vi "IMAQ FPGA Image Transfer from Target U8.vi"(6 "Image Transfer Size Alignment":u32(ring)=1 items=["1 Pixel"=1, "8 Pixels"=8, "16 Pixels"=16, "32 Pixels"=32], 7 "Read Timeout (ms)":i32=5000, 8 "error in (no error)":errorcluster, 9 "DMA FIFO Reference In":refnum<k20>, 10 "Maximum Pixels per Read":i32=-1, 11 "Image":T1) -> (0 "error out":errorcluster, 1 "DMA FIFO Reference Out":refnum<k20>, 3 "Image Out":T1)   [LabVIEW 2020, in "NI_VDM_FPGA_Basics.lvlib"]
doc: "Transfers an image from the target FPGA to the host processor via DMA FIFO."
uses:
  <vilib>/visionFPGA/NI_VDM_FPGA_Basics.lvlib
  <vilib>/vision/Image Controls.llb/IMAQ Image.ctl
  <vilib>/rvi/errors/niLvFpgaAdjustHostInterfaceError.vi
  <vilib>/rvi/interface/nirviMethod/nirviMethod.xnode
  <vilib>/FPGAPlugInAG/Dynamic/niLvFpga_ReadFifo_Dynamic.vi
  <vilib>/rvi/errors/niLvFpgaMergeErrorWithErrorCode.vi
  <vilib>/vision/EDVR.llb/IMAQ ImageToEDVR 2D U8.vi
  <vilib>/FPGAPlugInAG/Dynamic/niLvFpga_AcquireReadRegionFifo_Dynamic.vi
  nivissvc.dll
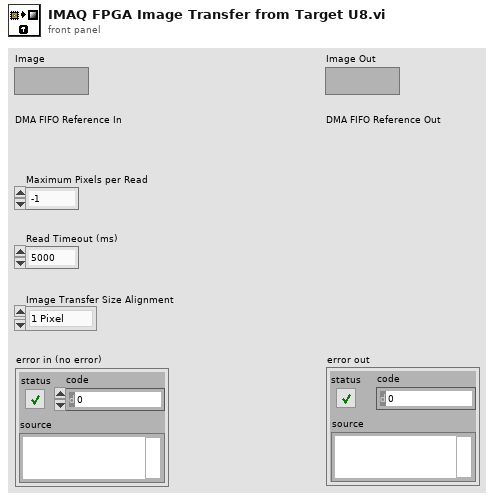
[diagram p1: front panel]
types:
  T1 = typedef "IMAQ Image.ctl" = refnum<image>
  T2 = typedef "Image Type" = u32
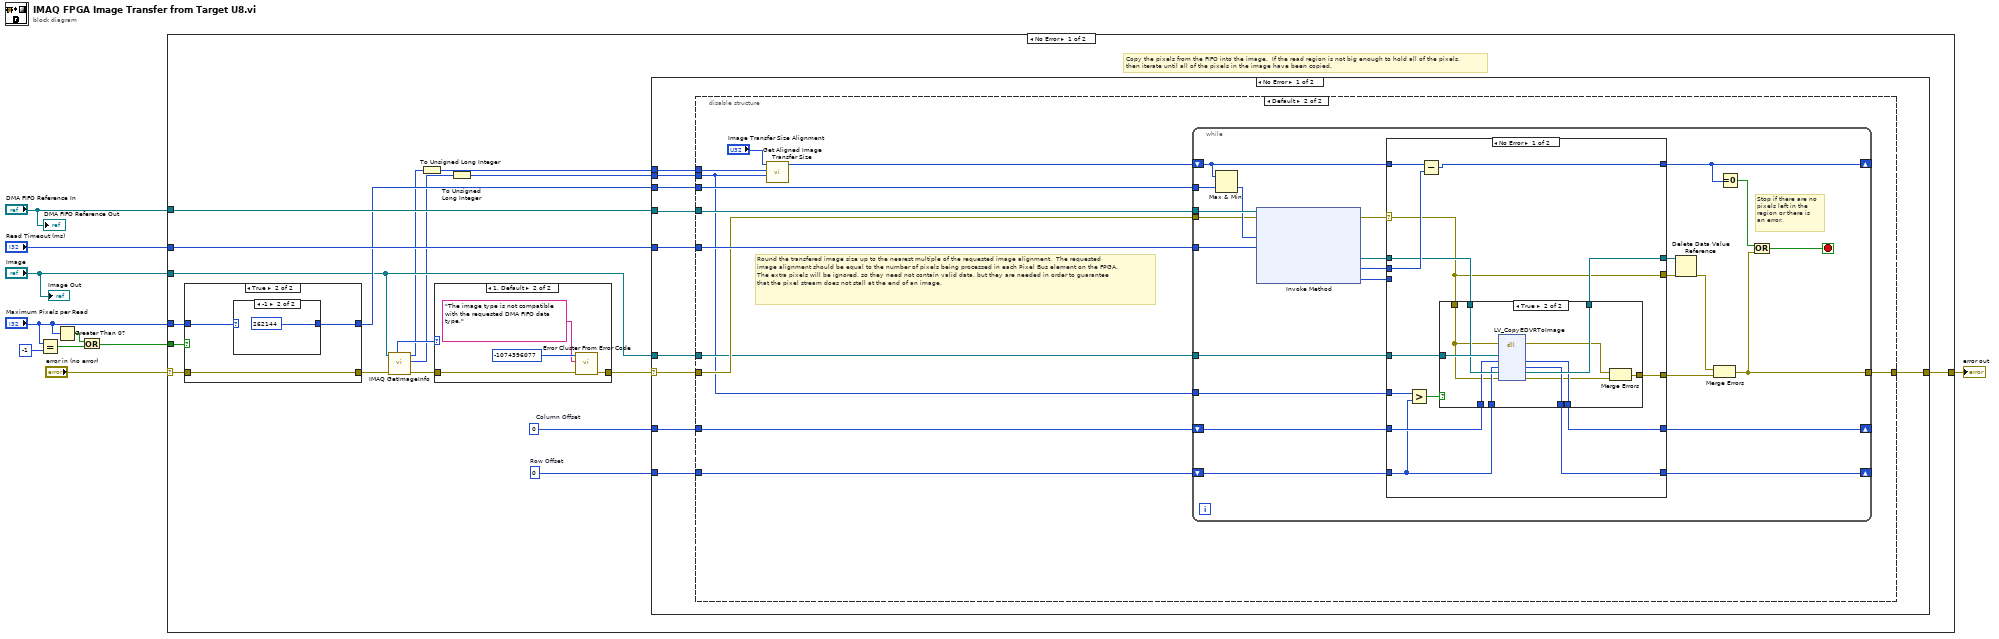
[diagram p0: block diagram]
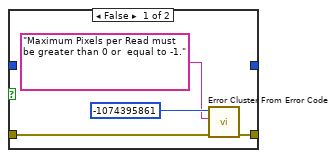
[diagram p2: hidden frame]
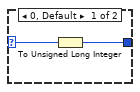
[diagram p3: hidden frame]
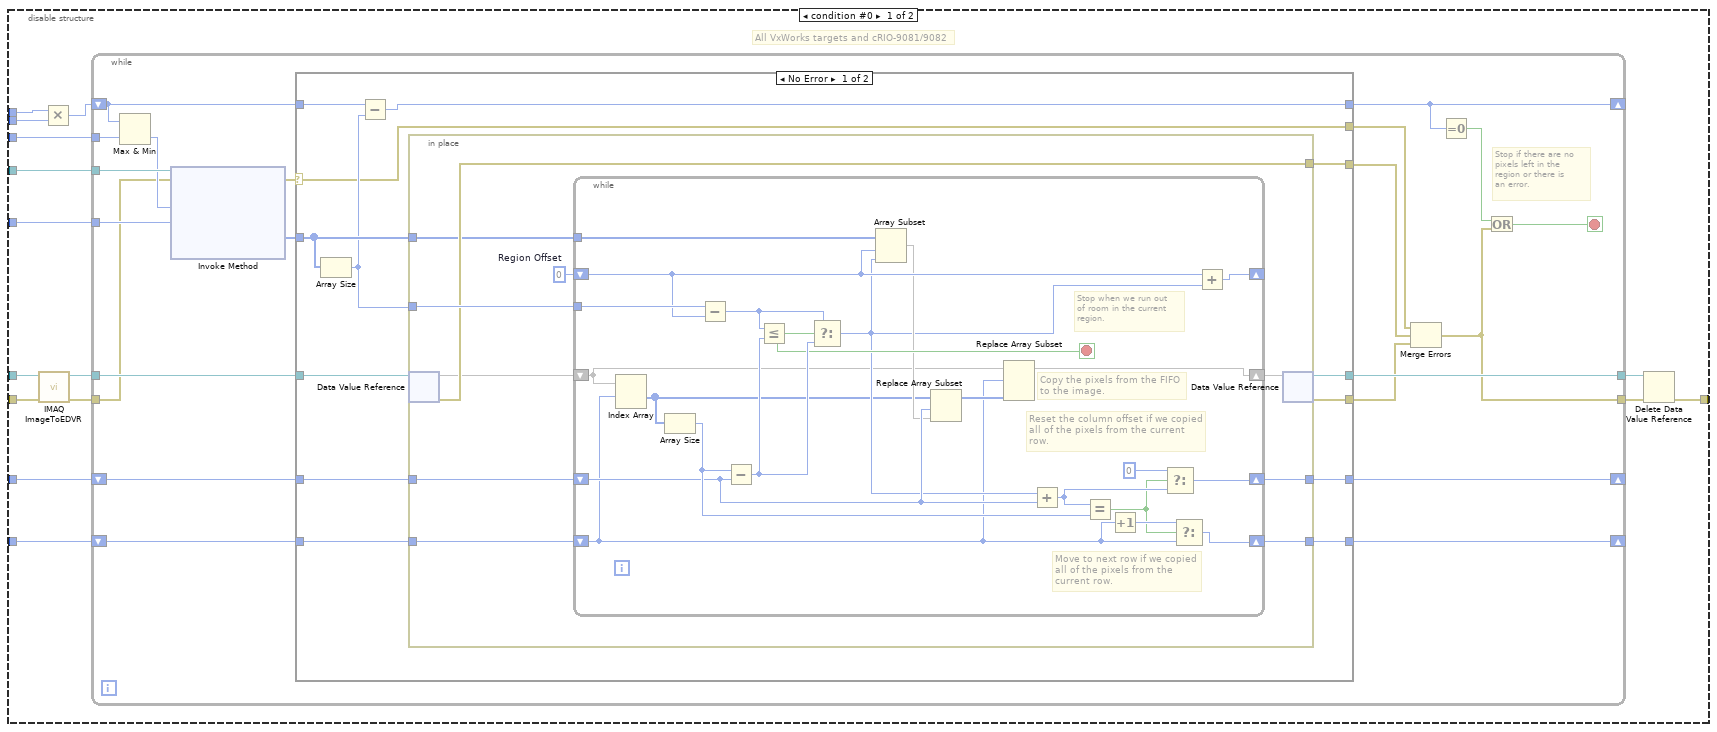
[diagram p5: hidden frame]
diagram:
  n1 = Equal?(x="Maximum Pixels per Read", y=-1) -> (x = y?=w6:bool)
  n2 = Greater Than 0?(x="Maximum Pixels per Read") -> (x > 0?=w7:bool)
  n3 = Or(x=w7, y=w6) -> (x .or. y?=w5:bool)
  n4 = case shown="No Error" "error in (no error)" {
    selector: "error in (no error)" -> [w15 w211]
    tunnel: "DMA FIFO Reference In" -> [w26 _]
    tunnel: "Read Timeout (ms)" -> [w23 _]
    tunnel: w5 -> [w22 _]
    tunnel: "Maximum Pixels per Read" -> [w21 _]
    tunnel: "Image" -> [w17 _]
    tunnel: [w16 w211] -> w2
    frame No Error {
      w27 = u32 0  # Row Offset
      w28 = u32 0  # Column Offset
      # "Copy the pixels from the FIFO into the image.  If the read region is not big enough to hold all of the pixels,\nthen iterate until all of the pixels in the image have been copied."
      n5 = case shown="True" w22 {
        tunnel: w15 -> [w30 w35]
        tunnel: [w29 w35] -> w20
        tunnel: w21 -> [_ w34]
        tunnel: [_ w33] -> w19
        frame False {
          n6 = call <vilib>:"Error Cluster From Error Code.vi"("error in (no error)"=w30, "error message (\"\")"="Maximum Pixels per Read must be greater than 0 or  equal to -1." ("error message (\"\")"), "error code (0)"=-1074395861) -> ("error out"=w29:errorcluster)  [unwired: 6 in]
        }
        frame True {
          n7 = case shown="-1" w34 {
            selector: w34 -> [w37 _]
            tunnel: [w36 u32 262144 ("Maximum Pixels per Write")] -> w33
            frame 0, Default {
              n8 = To Unsigned Long Integer(number=w37) -> (unsigned 32bit integer=w36:u32)
            }
            frame -1 {
            }
          }
        }
      }
      n9 = call "IMAQ GetImageInfo"("error in (no error)"=w20, "Image"=w17) -> ("error out"=w24:errorcluster, "Y Resolution"=w13:i32, "X Resolution"=w14:i32, "Image Type"=w25:T2)  [unwired: 2 in, 4 out]
      n10 = To Unsigned Long Integer(number=w14) -> (unsigned 32bit integer=w12:u32)
      n11 = case shown="1, Default" w25 {
        tunnel: w24 -> [w39 w41]
        tunnel: [w39 w40] -> w18
        frame 0 {
          # "Allowed types are:\nGrayscale (U8)"
        }
        frame 1, Default {
          n12 = call <vilib>:"Error Cluster From Error Code.vi"("error in (no error)"=w41, "error message (\"\")"="The image type is not compatible with the requested DMA FIFO data type." ("error message (\"\")"), "error code (0)"=-1074396077) -> ("error out"=w40:errorcluster)  [unwired: 6 in]
        }
      }
      n13 = To Unsigned Long Integer(number=w13) -> (unsigned 32bit integer=w11:u32)
      n14 = case shown="No Error" w18 {
        selector: w18 -> [w52 w210]
        tunnel: w28 -> [w51 _]
        tunnel: w27 -> [w50 _]
        tunnel: w26 -> [w48 _]
        tunnel: [w46 w210] -> w16
        tunnel: w19 -> [w47 _]
        tunnel: w23 -> [w49 _]
        tunnel: w17 -> [w53 _]
        tunnel: w12 -> [w45 _]
        tunnel: w11 -> [w44 _]
        frame No Error {
          n15 = disable-structure shown="Default" {
            disable-tunnel: w51 -> [w68 w151]
            disable-tunnel: w50 -> [w67 w150]
            disable-tunnel: w48 -> [w66 w149]
            disable-tunnel: [w57 w148] -> w46
            disable-tunnel: w47 -> [w65 w147]
            disable-tunnel: w49 -> [w64 w146]
            disable-tunnel: w53 -> [w63 w144]
            disable-tunnel: w52 -> [w61 w145]
            disable-tunnel: w45 -> [w55 w141]
            disable-tunnel: w44 -> [w54 w140]
            frame condition #0 {
              # "All VxWorks targets and cRIO-9081/9082"
              n16 = call-poly <vilib>:"IMAQ ImageToEDVR.vi"("error in (no error)"=w61, "Image"=w63) -> ("error out"=w60:errorcluster, "EDVR 2D U8"=w62:refnum<data-value>)  [unwired: 7 in, 1 out]
              n17 = Multiply(x=w55, y=w54) -> (x*y=w56:u32)
              n18 = while {
                shift-right: [w80] -> _
                shift-left: w56 -> [w76]
                shift-right: [w85] -> _
                shift-left: w68 -> [w87]
                shift-right: [w88] -> _
                shift-left: w67 -> [w86]
                tunnel: w66 -> [w84]
                tunnel: [w82] -> w59
                tunnel: [w78] -> w58
                tunnel: w65 -> [w74]
                tunnel: w64 -> [w73]
                tunnel: w62 -> [w70]
                tunnel: w60 -> [w69]
                stop <- w79 stop-if-true
                # "Stop if there are no\npixels left in the \nregion or there is\nan error."
                n19 = Max & Min(x=w76, y=w74) -> (min(x,y)=w75:u32)  [unwired: 1 out]
                n20 = xnode "Invoke Method"("FPGA VI Reference In"=w84, "error in"=w69, "Number of Elements"=w75, "Timeout (ms)"=w73) -> ("error out"=w83:errorcluster, "Data"=w89:u8[])  [unwired: 2 out]
                n21 = case shown="No Error" w83 {
                  selector: w83 -> [w90 w135]
                  tunnel: w76 -> [w102 w138]
                  tunnel: [w101 w138] -> w80
                  tunnel: w70 -> [w100 w139]
                  tunnel: w89 -> [w92 _]
                  tunnel: [w99 w136] -> w88
                  tunnel: w87 -> [w98 w137]
                  tunnel: w86 -> [w97 w136]
                  tunnel: [w96 w137] -> w85
                  tunnel: [w95 w139] -> w82
                  tunnel: [w90 w135] -> w72
                  tunnel: [w94 _] -> w71
                  tunnel: [w93 _] -> w81
                  frame No Error {
                    n22 = Array Size(array=w92) -> (size(s)=w91:i32)
                    n23 = Subtract(x=w102, y=w91) -> (x-y=w101:u32)
                    n24 = in-place {
                      in-place-border: w91 -> [w110]
                      in-place-border: [w112] -> w99
                      in-place-border: w98 -> [w109]
                      in-place-border: w97 -> [w105]
                      in-place-border: [w108] -> w96
                      in-place-border: [w107] -> w93
                      in-place-border: w92 -> [w103]
                      w111 = u32 0  # Region Offset
                      n25 = in-place-dvr #1(w100) -> (w106:u8[][], w107:errorcluster)
                      n26 = while {
                        shift-right: [w132] -> _
                        shift-left: w111 -> [w131]
                        tunnel: w103 -> [w121]
                        tunnel: w110 -> [w134]
                        shift-right: [w126] -> w108
                        shift-left: w109 -> [w122]
                        shift-right: [w113] -> w104
                        shift-left: w106 -> [w116]
                        shift-right: [w124] -> w112
                        shift-left: w105 -> [w114]
                        stop <- w123 stop-if-true
                        # "Stop when we run out\nof room in the current\nregion."
                        # "Copy the pixels from the FIFO\nto the image."
                        # "Reset the column offset if we copied\nall of the pixels from the current\nrow."
                        # "Move to next row if we copied\nall of the pixels from the\ncurrent row."
                        n27 = Index Array(array=w116, index (row)=w114) -> (element=w117:u8[])  [unwired: 1 in]
                        n28 = Array Size(array=w117) -> (size(s)=w130:i32)
                        n29 = Subtract(x=w134, y=w131) -> (x-y=w133:u32)
                        n30 = Subtract(x=w130, y=w122) -> (x-y=w129:u32)
                        n31 = Less Or Equal?(x=w133, y=w129) -> (x <= y?=w123:bool)
                        n32 = Select(t=w133, s=w123, f=w129) -> (s? t:f=w119:u32)
                        n33 = Array Subset(array=w121, index=w131, length=w119) -> (w120:u8[])
                        n34 = Replace Array Subset(array=w117, new element=w120, index=w122) -> (w115:u8[])
                        n35 = Replace Array Subset(array=w116, new element=w115, index (row)=w114) -> (w113:u8[][])  [unwired: 1 in]
                        n36 = Add(x=w119, y=w122) -> (x+y=w127:u32)
                        n37 = Equal?(x=w127, y=w130) -> (x = y?=w118:bool)
                        n38 = Increment(x=w114) -> (x+1=w125:u32)
                        n39 = Select(t=u32 0 ("Elements In Region"), s=w118, f=w127) -> (s? t:f=w126:u32)
                        n40 = Select(t=w125, s=w118, f=w114) -> (s? t:f=w124:u32)
                        n41 = Add(x=w131, y=w119) -> (x+y=w132:u32)
                      }
                      n42 = in-place-dvr #1(w104) -> (w95:refnum<data-value>, w94:errorcluster)
                    }
                  }
                  frame Error {
                  }
                }
                n43 = Merge Errors(w72, w81, w71) -> (w78:errorcluster)
                n44 = Equal To 0?(x=w80) -> (x = 0?=w77:bool)
                n45 = Or(x=w77, y=w78) -> (x .or. y?=w79:bool)
              }
              n46 = Delete Data Value Reference(data value reference=w59, error in=w58) -> (error out=w57:errorcluster)  [unwired: 1 out]
            }
            frame condition #1 (active) {
              # "Round the transfered image size up to the nearest multiple of the requested image alignment.  The requested image alignment should be equal to the number of pixels being processed in each Pixel Bus element on the FPGA.  The extra pixels will be ignored, so they need not contain valid data, but they are needed in order to guarantee that the pixel stream does not stall at the end of an image."
              n47 = call <vilib>:"Get Aligned Image Transfer Size.vi"("Y Resolution"=w140, "X Resolution"=w141, "Image Transfer Size Alignment"="Image Transfer Size Alignment") -> ("Aligned Image Transfer Size"=w142:u64)  [unwired: 8 in]
              n48 = while {
                shift-right: [w166] -> _
                shift-left: w142 -> [w163]
                shift-right: [w170] -> _
                shift-left: w151 -> [w172]
                shift-right: [w173] -> _
                shift-left: w150 -> [w171]
                tunnel: w149 -> [w169]
                tunnel: [w153] -> w148
                tunnel: w147 -> [w160]
                tunnel: w146 -> [w159]
                tunnel: w145 -> [w158]
                tunnel: w144 -> [w157]
                tunnel: w140 -> [w152]
                stop <- w165 stop-if-true
                # "Stop if there are no\npixels left in the \nregion or there is\nan error."
                n49 = Max & Min(x=w163, y=w160) -> (min(x,y)=w162:u64)  [unwired: 1 out]
                n50 = xnode "Invoke Method"("FPGA VI Reference In"=w169, "error in"=w158, "Number of Elements"=w162, "Timeout (ms)"=w159) -> ("error out"=w168:errorcluster, "Read Region Reference"=w175:refnum<data-value>, "Elements In Region"=w174:u32, "Elements Remaining"=w161:u32)  [unwired: 1 out]
                n51 = case shown="No Error" w168 {
                  selector: w168 -> [w179 w205]
                  tunnel: w163 -> [w189 w209]
                  tunnel: [w188 w209] -> w166
                  tunnel: w175 -> [w184 w206]
                  tunnel: w174 -> [w185 _]
                  tunnel: [w181 w207] -> w173
                  tunnel: w172 -> [w183 w208]
                  tunnel: w171 -> [w177 w207]
                  tunnel: [w182 w208] -> w170
                  tunnel: [w186 w206] -> w167
                  tunnel: [w179 w205] -> w156
                  tunnel: w161 -> [_ _]
                  tunnel: w157 -> [w187 _]
                  tunnel: [w180 w205] -> w155
                  tunnel: w152 -> [w176 _]
                  frame No Error {
                    n52 = Greater?(x=w176, y=w177) -> (0:w178:bool)
                    n53 = Subtract(x=w189, y=w185) -> (x-y=w188:u64)
                    n54 = case shown="True" w178 {
                      tunnel: w187 -> [_ w204]
                      tunnel: [w192 w203] -> w186
                      tunnel: w184 -> [w192 w202]
                      tunnel: w183 -> [w190 w201]
                      tunnel: w177 -> [w191 w200]
                      tunnel: [w190 w199] -> w182
                      tunnel: [w191 w198] -> w181
                      tunnel: [w193 w195] -> w180
                      tunnel: w179 -> [w193 w194]
                      frame False {
                      }
                      frame True {
                        n55 = dll-call lib="nivissvc.*" fn="LV_CopyEDVRToImage"(error in=w194, "image"=w204, "xImageOffset"=w201, "yImageOffset"=w200, "EDVR"=w202, "error"=w194) -> (error out=w196:errorcluster, "xImageOffset"=w199:u32, "yImageOffset"=w198:u32, "EDVR"=w203:refnum<data-value>, "error"=w197:errorcluster)  [unwired: 4 in, 1 out]
                        n56 = Merge Errors(w196, w197) -> (w195:errorcluster)
                      }
                    }
                  }
                  frame Error {
                  }
                }
                n57 = Delete Data Value Reference(data value reference=w167, error in=w156) -> (error out=w154:errorcluster)  [unwired: 1 out]
                n58 = Merge Errors(w154, w155) -> (w153:errorcluster)
                n59 = Equal To 0?(x=w166) -> (x = 0?=w164:bool)
                n60 = Or(x=w164, y=w153) -> (x .or. y?=w165:bool)
              }
            }
          }
        }
        frame Error {
        }
      }
    }
    frame Error {
    }
  }
  "error out" <- w2
  "Image Out" <- "Image"
  "DMA FIFO Reference Out" <- "DMA FIFO Reference In"
